vi "Epoch Factory.vi"(11 "Epoch (Local System)":T1) -> (3 "Epoch object":refnum<class "Epoch.lvclass">)   [LabVIEW 2013]
uses:
  epoch/Epoch.lvclass
  Epochs -- enum.ctl
  epoch.UTC/Epoch.UTC.lvclass
  epoch.UNIX/Epoch.UNIX.lvclass
  epoch.GPS/Epoch.GPS.lvclass
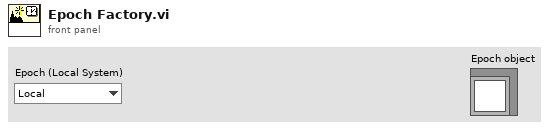
[diagram p1: front panel]
types:
  T1 = typedef "Epochs -- enum.ctl" = enum16{"Local", "UTC", "Unix", "GPS"}
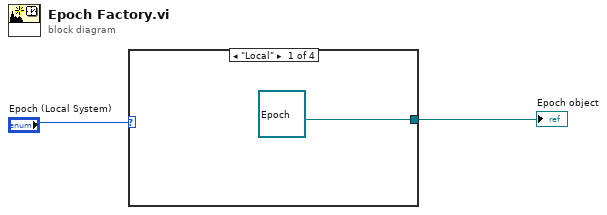
[diagram p0: block diagram]
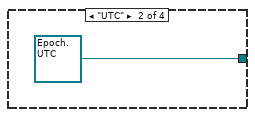
[diagram p2: hidden frame]
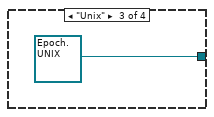
[diagram p3: hidden frame]
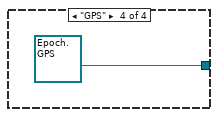
[diagram p4: hidden frame]
diagram:
  n1 = case shown="\"Local\"" "Epoch (Local System)" {
    tunnel: [refnum<class "Epoch.lvclass"> refnum ("Epoch.lvclass") refnum<class "Epoch.UTC.lvclass"> refnum ("Epoch.UTC.lvclass") refnum<class "Epoch.UNIX.lvclass"> refnum ("Epoch.UNIX.lvclass") refnum<class "Epoch.GPS.lvclass"> refnum ("Epoch.GPS.lvclass")] -> w1
    frame "Local" {
    }
    frame "UTC" {
    }
    frame "Unix" {
    }
    frame "GPS" {
    }
  }
  "Epoch object" <- w1
